vi "Main.vi"() -> ()   [LabVIEW 2022 SP3]
uses:
  ctrls/Shared_Image.ctl
  02808b36-664e-4593-b76e-2143e1b1c9f3.vi
  c9e93c7d-3384-4800-9441-c92ed6a90da8.vi
panel:
  in  "Script Flag":bool
  out "Script Connected":bool
  in  "Stop":bool
  in  "Single Action":bool
  in  "Continuous Action":bool
  in  "Timeout T [ms]":i32=50
  out "Current Event":string
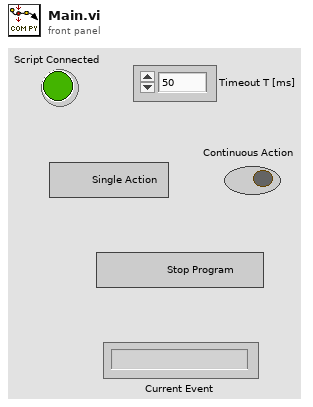
[diagram p1: front panel]
types:
  T1 = typedef "Shared_Image.ctl" = cluster{"Updated":bool, "2D Image":dbl[][]}
  T2 = enum8{"Enabled", "Disabled", "Disabled and Grayed Out"}
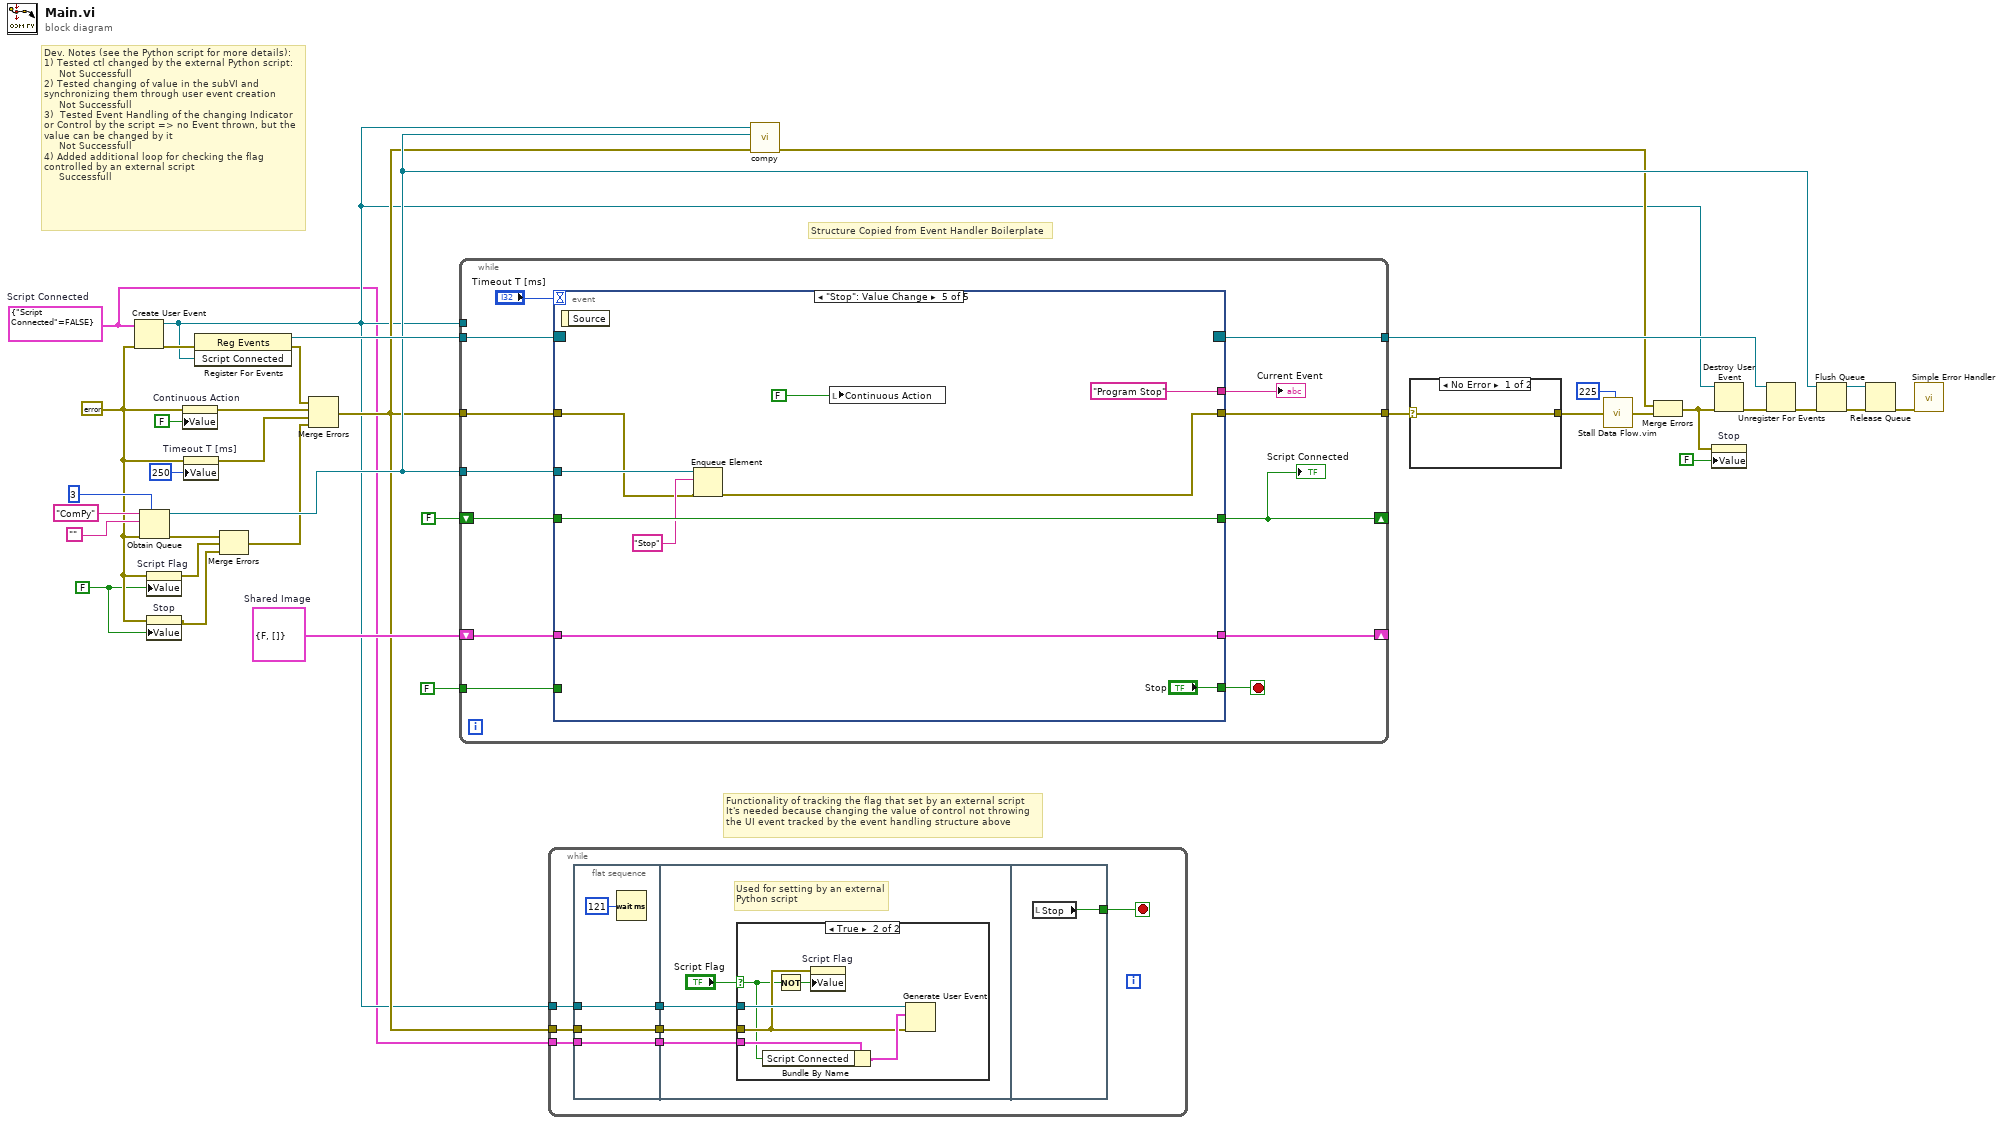
[diagram p0: block diagram]
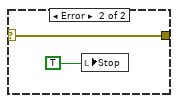
[diagram p2: hidden frame]
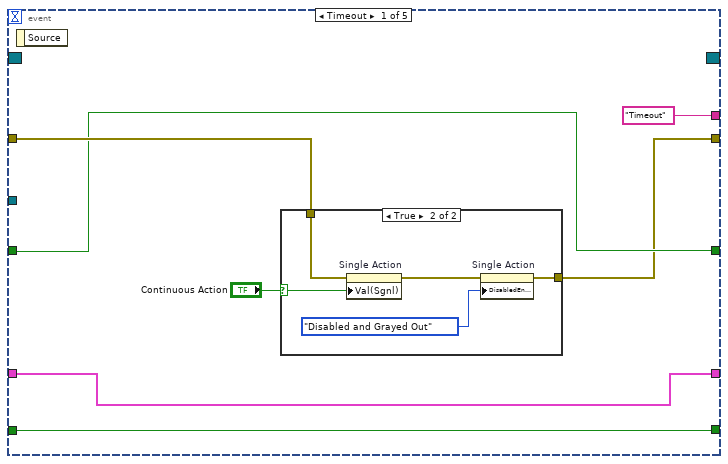
[diagram p4: hidden frame]
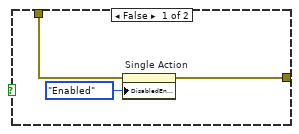
[diagram p5: hidden frame]
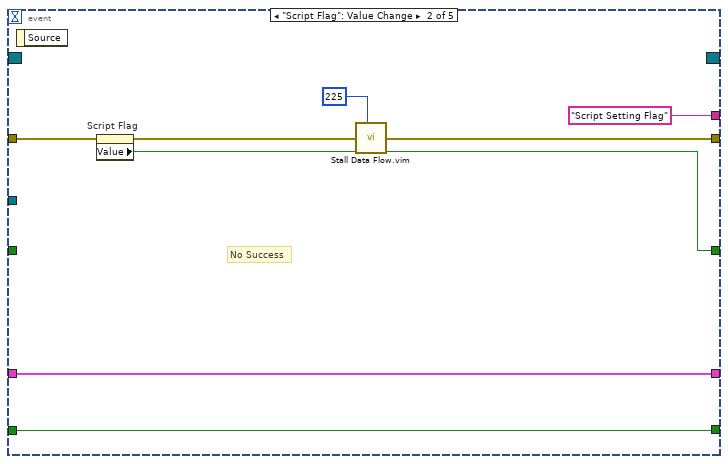
[diagram p6: hidden frame]
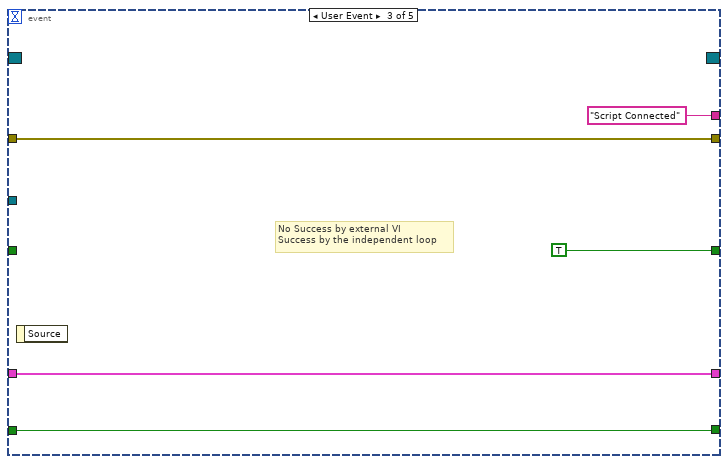
[diagram p7: hidden frame]
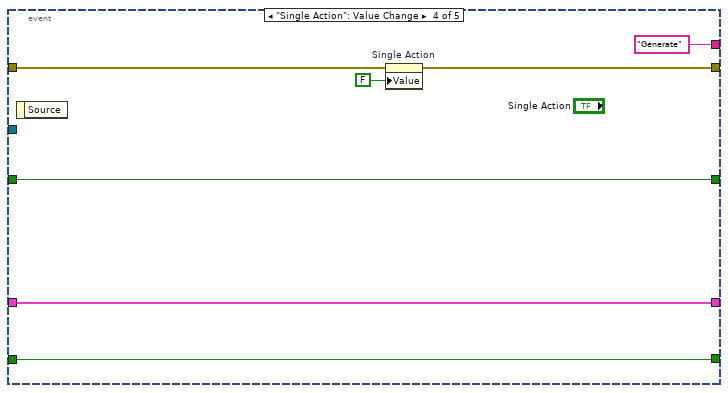
[diagram p8: hidden frame]
diagram:
  w7 = FALSE ("Script Flag")
  w10 = cluster{"Script Connected":bool} {"Script Connected"=FALSE}  # Script Connected
  w31 = T1 {"Updated"=FALSE, "2D Image"=[]}  # Shared Image
  w8 = errorcluster {"status"=FALSE, "code"=0, "source"=""} ("error in (no error)")
  # "Functionality of tracking the flag that set by an external script\nIt's needed because changing the value of control not throwing\nthe UI event tracked by the event handling structure above"
  # "Dev. Notes (see the Python script for more details):\n1) Tested ctl changed by the external Python script:\n     Not Successfull\n2) Tested changing of value in the subVI and \nsynchronizing them through user event creation\n     Not Successfull\n3)  Tested Event Handling of the changing Indicator \nor Control by the script => no Event thrown, but the\nvalue can be changed by it\n     Not Successfull\n4) Added additional loop for checking the flag\ncontrolled by an external script\n     Successfull"
  # "Structure Copied from Event Handler Boilerplate"
  n1 = Create User Event(user event datatype=w10, error in=w8) -> (user event=w11:refnum<user-event>, error out=w30:errorcluster)
  n2 = Obtain Queue(max queue size (-1, unlimited)=3, name (unnamed)="ComPy", element data type="", error in (no error)=w8) -> (queue out=w18:refnum<queue>, error out=w16:errorcluster)  [unwired: 1 in, 1 out]
  n3 = property on="Script Flag" class="Bool (strict)"(error in=w8, "Value"=w7) -> (error out=w15:errorcluster)  [unwired: 1 in, 1 out]
  n4 = property on="Stop" class="Bool (strict)"(error in=w8, "Value"=w7) -> (error out=w6:errorcluster)  [unwired: 1 in, 1 out]
  n5 = property on="Continuous Action" class="Bool (strict)"(error in=w8, "Value"=FALSE ("Continuous Generation")) -> (error out=w35:errorcluster)  [unwired: 1 in, 1 out]
  n6 = property on="Timeout T [ms]" class="DigNum (strict)"(error in=w8, "Value"=250 ("Timeout")) -> (error out=w34:errorcluster)  [unwired: 1 in, 1 out]
  n7 = register-events(error in=w30, w11) -> (reference out=w28:refnum<event-registration>, error out=w29:errorcluster)  [unwired: 1 in]
  n8 = Merge Errors(w16, w15, w6) -> (w14:errorcluster)
  n9 = Merge Errors(w29, w35, w34, w14) -> (w12:errorcluster)
  n10 = while {
    tunnel: FALSE ("Generate") -> [w47]
    tunnel: w12 -> [w45]
    shift-right: [w43] -> _
    shift-left: w31 -> [w44]
    shift-right: [w37] -> _
    shift-left: FALSE ("Value") -> [w42]
    tunnel: [w41] -> w9
    tunnel: w28 -> [w40]
    tunnel: [w39] -> w27
    tunnel: w18 -> [w38]
    tunnel: w11 -> [_]
    stop <- w48 stop-if-true
    n11 = event shown="[4] \"Stop\": Value Change" {
      selector: w40 -> [_ _ _ _ _]
      dyn-events: [_ _ _ _ _] -> w39
      timeout: "Timeout T [ms]" -> [_ _ _ _ _]
      tunnel: [w56 w72 w75 w83 "Stop"] -> w48
      tunnel: w47 -> [w56 w72 w75 w83 _]
      tunnel: ["Timeout" ("State") "Script Setting Flag" ("State") "Script Connected" ("State") "Generate" ("State") "Program Stop" ("State")] -> w46
      tunnel: w45 -> [w53 w70 w77 w80 w86]
      tunnel: w44 -> [w52 w71 w74 w82 w90]
      tunnel: [w52 w71 w74 w82 w90] -> w43
      tunnel: w42 -> [w51 _ _ w81 w89]
      tunnel: [w51 w69 TRUE w81 w89] -> w37
      tunnel: [w50 w66 w77 w78 w85] -> w41
      tunnel: w38 -> [_ _ _ _ w88]
      event Timeout {
        n12 = event-data() -> ()  [unwired: 1 in, 1 out]
        n13 = case shown="True" "Continuous Action" {
          selector: "Continuous Action" -> [_ w63]
          tunnel: w53 -> [w59 w64]
          tunnel: [w57 w60] -> w50
          frame False {
            n14 = property on="Single Action" class="Bool (strict)"(error in=w59, "DisabledEnum"=T2."Enabled" ("Disabled")) -> (error out=w57:errorcluster)  [unwired: 1 in, 1 out]
          }
          frame True {
            n15 = property on="Single Action" class="Bool (strict)"(error in=w64, "Val(Sgnl)"=w63) -> (error out=w62:errorcluster)  [unwired: 1 in, 1 out]
            n16 = property on="Single Action" class="Bool (strict)"(error in=w62, "DisabledEnum"=T2."Disabled and Grayed Out" ("Disabled")) -> (error out=w60:errorcluster)  [unwired: 1 in, 1 out]
          }
        }
      }
      event "Script Flag": Value Change {
        # "No Success"
        n17 = event-data() -> ()  [unwired: 1 in, 1 out]
        n18 = property on="Script Flag" class="Bool (strict)"(error in=w70) -> (error out=w67:errorcluster, "Value"=w69:bool)  [unwired: 1 in, 1 out]
        n19 = call "Stall Data Flow.vim"("value in"=w67, "milliseconds to wait"=u32 225) -> ("value out"=w66:errorcluster)  [unwired: 1 out]
      }
      event User Event {
        # "No Success by external VI\nSuccess by the independent loop"
        n20 = event-data() -> ()  [unwired: 1 in, 1 out]
      }
      event "Single Action": Value Change {
        n21 = event-data() -> ()  [unwired: 1 in, 1 out]
        n22 = property on="Single Action" class="Bool (strict)"(error in=w80, "Value"=FALSE ("Single Action")) -> (error out=w78:errorcluster)  [unwired: 1 in, 1 out]
      }
      event "Stop": Value Change {
        n23 = event-data() -> ()  [unwired: 1 in, 1 out]
        n24 = Enqueue Element(queue=w88, element="Stop", error in (no error)=w86) -> (error out=w85:errorcluster)  [unwired: 1 in, 2 out]
        n25 = local write "Continuous Action"(FALSE ("Timeout Generation")) -> ()
      }
    }
    "Current Event" <- w46
    "Script Connected" <- w37
  }
  n26 = while {
    tunnel: w12 -> [w99]
    tunnel: w11 -> [w96]
    tunnel: w10 -> [w94]
    stop <- w100 stop-if-true
    n27 = flat-sequence {
      tunnel: w99 -> [w103]
      tunnel: [w103] -> w98
      tunnel: [w102] -> w97
      tunnel: w96 -> [w102]
      tunnel: w94 -> [w101]
      tunnel: [w101] -> w95
      tunnel: w98 -> [w107]
      tunnel: w97 -> [w106]
      tunnel: w95 -> [w105]
      tunnel: [w115] -> w100
      frame #0 {
        n28 = Wait (ms)(milliseconds to wait=u32 121) -> ()  [unwired: 1 out]
      }
      frame #1 {
        # "Used for setting by an external\nPython script"
        n29 = case shown="True" "Script Flag" {
          selector: "Script Flag" -> [_ w110]
          tunnel: w107 -> [_ w111]
          tunnel: w106 -> [_ w114]
          tunnel: w105 -> [_ w113]
          frame False {
          }
          frame True {
            n30 = Bundle By Name(cluster=w113, "Script Connected"=w110) -> (w112:cluster{"Script Connected":bool})
            n31 = Not(x=w110) -> (.not. x?=w109:bool)
            n32 = property on="Script Flag" class="Bool (strict)"(error in=w111, "Value"=w109) -> ()  [unwired: 1 in, 2 out]
            n33 = Generate User Event(user event=w114, event data cluster=w112, error in=w111) -> ()  [unwired: 1 in, 2 out]
          }
        }
      }
      frame #2 {
        n34 = local read "Stop"() -> (w115:bool)
      }
    }
  }
  n35 = call "compy.vi"("error in"=w12, "Commands Queue"=w18, "User Event Ref IN"=w11) -> ("error out"=w17:errorcluster)  [unwired: 8 in]
  n36 = case shown="No Error" w9 {
    selector: w9 -> [w116 w117]
    tunnel: [w116 w117] -> w4
    frame No Error {
    }
    frame Error {
      n37 = local write "Stop"(TRUE ("Stop")) -> ()
    }
  }
  n38 = call "Stall Data Flow.vim"("value in"=w4, "milliseconds to wait"=u32 225) -> ("value out"=w3:errorcluster)  [unwired: 1 out]
  n39 = Merge Errors(w17, w3) -> (w2:errorcluster)
  n40 = property on="Stop" class="Bool (strict)"(error in=w2, "Value"=FALSE ("Stop")) -> ()  [unwired: 1 in, 2 out]
  n41 = Destroy User Event(user event=w11, error in=w2) -> (error out=w26:errorcluster)
  n42 = Unregister For Events(event registration refnum=w27, error in=w26) -> (error out=w22:errorcluster)
  n43 = Flush Queue(queue=w18, error in (no error)=w22) -> (queue out=w20:refnum<queue>, error out=w21:errorcluster)  [unwired: 1 out]
  n44 = Release Queue(queue=w20, error in (no error)=w21) -> (error out=w19:errorcluster)  [unwired: 1 in, 2 out]
  n45 = call <vilib>:"Simple Error Handler.vi"("error in (no error)"=w19) -> ()  [unwired: 4 in, 5 out]
